vi "LS4 SetMotorCurrent_SD.vi"(1 "Motor Currents":dbl[](array[numeric]), 2 "DLL path in":path) -> (0 "error out":errorcluster)   [LabVIEW 2016, in "DelayLineLS4.lvclass"]
uses:
  Classes/Delay Line/LS4/DelayLineLS4.lvclass
  <vilib>/ErrorRing/Error Ring.xnode
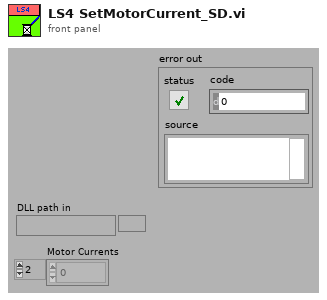
[diagram p1: front panel]
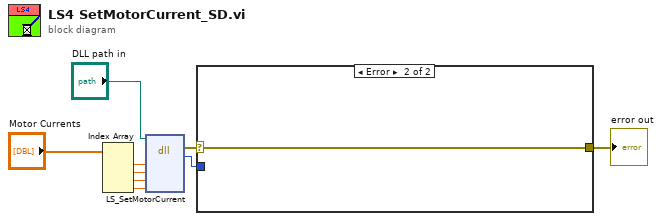
[diagram p0: block diagram]
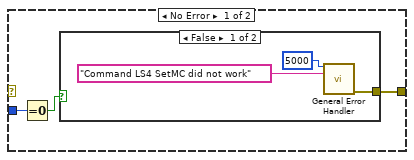
[diagram p2: hidden frame]
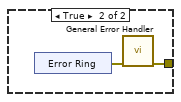
[diagram p3: hidden frame]
diagram:
  n1 = Index Array(array="Motor Currents") -> (element #1=w4:dbl, element #2=w3:dbl, element #3=w2:dbl, element #4=w1:dbl)  [unwired: 4 in]
  n2 = dll-call lib="S:/TRANCON/DLL/LStep4.dll" fn="LS_SetMotorCurrent"(path in="DLL path in", "X"=w4, "Y"=w3, "Z"=w2, "A"=w1) -> (error out=w6:errorcluster, "return type"=w9:i32)  [unwired: 6 in, 1 out]
  n3 = case shown="Error" w6 {
    selector: w6 -> [_ w19]
    tunnel: w9 -> [w12 _]
    tunnel: [w11 w19] -> w8
    frame No Error {
      n4 = Equal To 0?(x=w12) -> (x = 0?=w10:bool)
      n5 = case shown="False" w10 {
        tunnel: [w13 w16] -> w11
        frame False {
          n6 = call <vilib>:"General Error Handler.vi"("[error code] (0)"=5000 ("code"), "[error source] (\" \")"="Command LS4 SetMC did not work" ("String to Prepend to source (\"\")")) -> ("error out"=w13:errorcluster)  [unwired: 9 in, 4 out]
        }
        frame True {
          n7 = xnode "Error Ring"() -> ("error out"=w17:errorcluster)
          n8 = call <vilib>:"General Error Handler.vi"("error in (no error)"=w17) -> ("error out"=w16:errorcluster)  [unwired: 10 in, 4 out]
        }
      }
    }
    frame Error {
    }
  }
  "error out" <- w8
